vi "IO_Fun.vi"(7 "DIO3232_Action":T2, 8 "error in (no error)":errorcluster, 11 "I/Oin":T1 {"Port" items=["input_port0", "input_port1", "input_port2", "input_port03", "output_port0", "output_port1", "output_port2", "output_port03"]; "Point" max=31}) -> (0 "error out":errorcluster, 3 "I/O out":T1 {"Port" items=["input_port0", "input_port1", "input_port2", "input_port03", "output_port0", "output_port1", "output_port2", "output_port03"]})   [LabVIEW 2014]
uses:
  Dio3232_controls.ctl
panel:
  # "input_port0  ÂI¦ìinput0~7\ninput_port1  ÂI¦ìinput8~15\ninput_port2  ÂI¦ìinput16~23\ninput_port3  ÂI¦ìinput24~31"
  # "output_port0  ÂI¦ìoutput0~7\noutput_port1  ÂI¦ìoutput8~15\noutput_port2  ÂI¦ìoutput16~23\noutput_port3  ÂI¦ìoutput24~31"
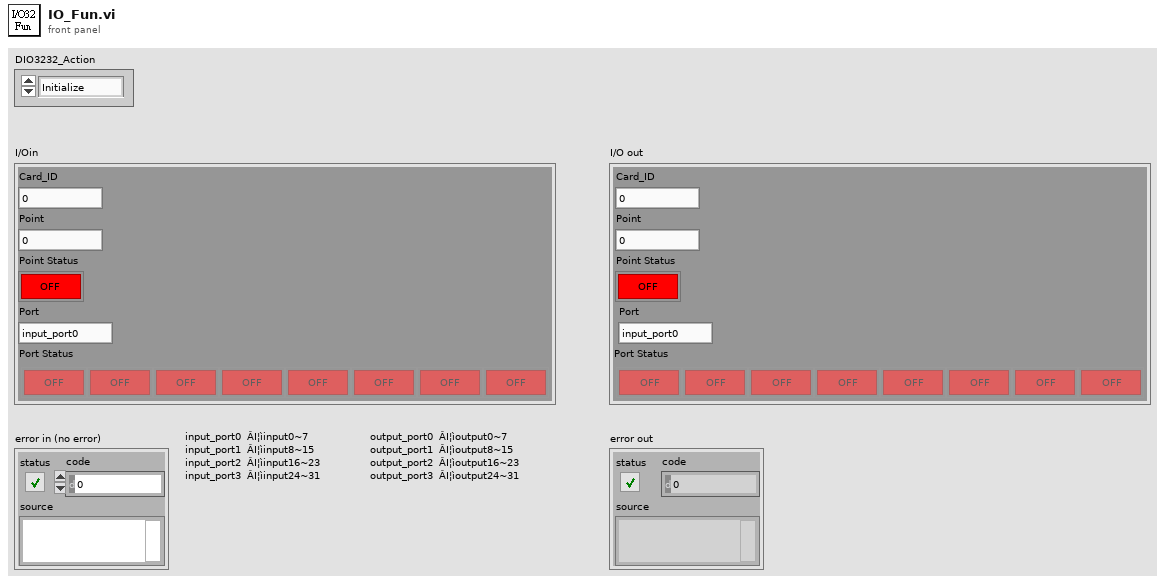
[diagram p1: front panel]
types:
  T1 = cluster{"Card_ID":u8, "Point":u16, "Point Status":bool, "Port":u8, "Port Status":bool[]}
  T2 = typedef "Dio3232_controls.ctl" = enum16{"Initialize", "read_in_point", "read_out_point", "read_port", "set_out_point", "set_port", "close", "Idle"}
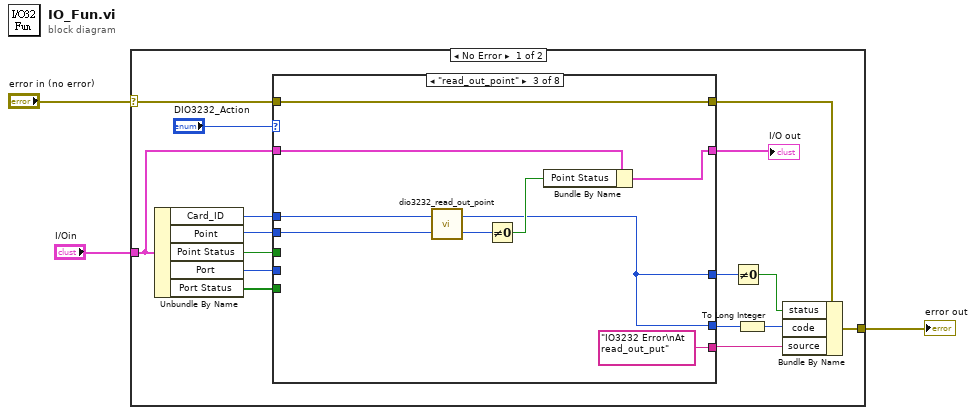
[diagram p0: block diagram]
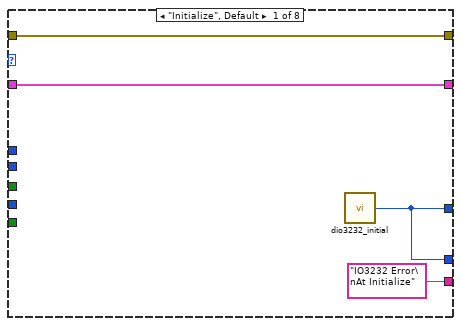
[diagram p2: hidden frame]
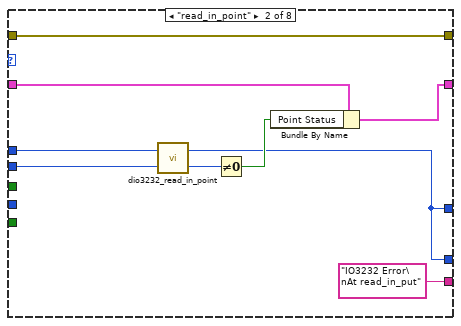
[diagram p3: hidden frame]
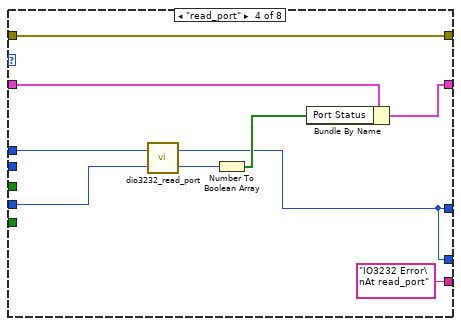
[diagram p4: hidden frame]
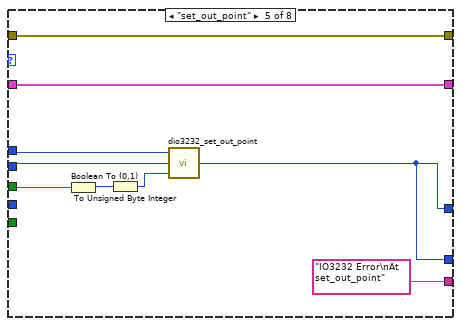
[diagram p5: hidden frame]
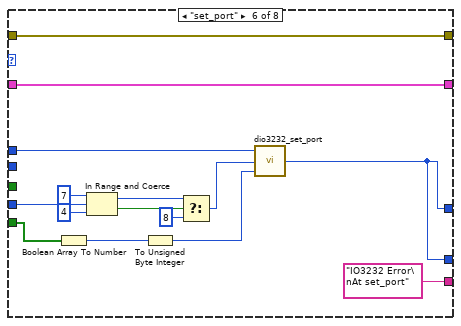
[diagram p6: hidden frame]
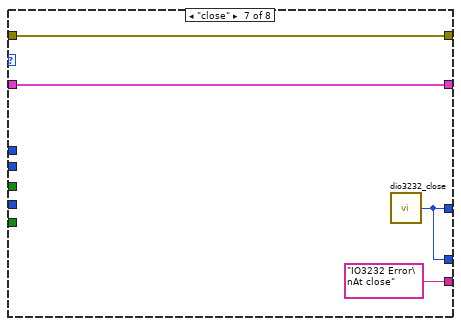
[diagram p7: hidden frame]
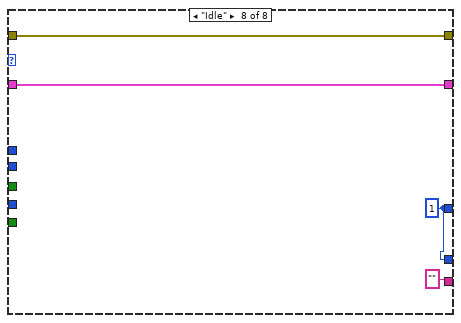
[diagram p8: hidden frame]
diagram:
  n1 = case shown="No Error" "error in (no error)" {
    selector: "error in (no error)" -> [w16 w83]
    tunnel: "I/Oin" -> [w18 _]
    tunnel: [w14 w83] -> w1
    frame No Error {
      n2 = Unbundle By Name(w18) -> ("Card_ID"=w13:u8, "Point"=w11:u16, "Point Status"=w7:bool, "Port"=w8:u8, "Port Status"=w6:bool[])
      n3 = case shown="\"read_out_point\"" "DIO3232_Action" {
        tunnel: w18 -> [w23 w29 w37 w46 w52 w73 w77 w81]
        tunnel: [w23 w28 w36 w45 w52 w73 w77 w81] -> w17
        tunnel: w16 -> [w22 w32 w41 w50 w59 w74 w78 w82]
        tunnel: [w22 w32 w41 w50 w59 w74 w78 w82] -> w15
        tunnel: w13 -> [_ w31 w40 w49 w58 w72 _ _]
        tunnel: [w20 w24 w33 w42 w51 w60 w75 w79] -> w10
        tunnel: ["IO3232 Error\nAt Initialize" "IO3232 Error\nAt read_in_put" "IO3232 Error\nAt read_out_put" "IO3232 Error\nAt read_port" "IO3232 Error\nAt set_out_point" "IO3232 Error\nAt set_port" "IO3232 Error\nAt close" ""] -> w12
        tunnel: w11 -> [_ w30 w39 _ w56 _ _ _]
        tunnel: w8 -> [_ _ _ w48 _ w71 _ _]
        tunnel: w7 -> [_ _ _ _ w55 _ _ _]
        tunnel: w6 -> [_ _ _ _ _ w70 _ _]
        tunnel: [w20 w24 w33 w42 w51 w60 w75 w79] -> w4
        frame "Initialize", Default {
          n4 = call "dio3232_initial.vi"() -> ("error_code"=w20:u32)
        }
        frame "read_in_point" {
          n5 = call "dio3232_read_in_point.vi"("Point"=w30, "CardID"=w31) -> ("State"=w27:u8, "error_code"=w24:u32)
          n6 = Not Equal To 0?(x=w27) -> (x != 0?=w26:bool)
          n7 = Bundle By Name(cluster=w29, "Point Status"=w26) -> (w28:T1)
        }
        frame "read_out_point" {
          n8 = call "dio3232_read_out_point.vi"("Point"=w39, "CardID"=w40) -> ("State"=w34:u8, "error_code"=w33:u32)
          n9 = Not Equal To 0?(x=w34) -> (x != 0?=w35:bool)
          n10 = Bundle By Name(cluster=w37, "Point Status"=w35) -> (w36:T1)
        }
        frame "read_port" {
          n11 = call "dio3232_read_port.vi"("Port"=w48, "CardID"=w49) -> ("Data"=w44:u8, "error_code"=w42:u32)
          n12 = Number To Boolean Array(number=w44) -> (Boolean array=w43:bool[])
          n13 = Bundle By Name(cluster=w46, "Port Status"=w43) -> (w45:T1)
        }
        frame "set_out_point" {
          n14 = Boolean To (0,1)(Boolean=w55) -> (0, 1=w54:i16)
          n15 = To Unsigned Byte Integer(number=w54) -> (unsigned 8bit integer=w53:u8)
          n16 = call "dio3232_set_out_point.vi"("State"=w53, "Point"=w56, "CardID"=w58) -> ("error_code"=w51:u32)
        }
        frame "set_port" {
          n17 = Boolean Array To Number(Boolean array=w70) -> (number=w69:u32)
          n18 = In Range and Coerce(upper limit=u8 7, x=w71, lower limit=u8 4) -> (coerced(x)=w62:u8, In Range?=w66:bool)
          n19 = To Unsigned Byte Integer(number=w69) -> (unsigned 8bit integer=w68:u8)
          n20 = Select(t=w62, s=w66, f=u8 8) -> (s? t:f=w61:u8)
          n21 = call "dio3232_set_port.vi"("Data"=w68, "Port"=w61, "CardID"=w72) -> ("error_code"=w60:u32)
        }
        frame "close" {
          n22 = call "dio3232_close.vi"() -> ("error_code"=w75:u32)
        }
        frame "Idle" {
          w79 = u32 1 ("error_code")
        }
      }
      "I/O out" <- w17
      n23 = Not Equal To 0?(x=w10) -> (x != 0?=w9:bool)
      n24 = To Long Integer(number=w4) -> (32bit integer=w5:i32)
      n25 = Bundle By Name(cluster=w15, "status"=w9, "code"=w5, "source"=w12) -> (w14:errorcluster)
    }
    frame Error {
    }
  }
  "error out" <- w1
